vi "Core Create.vi"(8 "error in (no error)":errorcluster, 10 "Plugin Name":string, 11 "CIFTemplateNode in":refnum<class "CIFCorePlugin.lvclass">) -> (0 "error out":errorcluster, 3 "CIFTemplateNode out":refnum<class "CIFCorePlugin.lvclass">)   [LabVIEW 2021, in "CIFCorePlugin.lvclass"]
uses:
  CIFCorePlugin.lvclass
  CIFCorePlugin.lvclass/CIFCorePlugin.ctl
  CIFCoreCommon/Typedef/Plugin State.ctl
  CIFCoreCommon/CIFCoreCommon.lvlib
  CIFCoreCommon/Typedef/Timing Stats Base.ctl
  CIFCoreCommon/Typedef/Timing Statistics.ctl
  CIFCoreCommon/Typedef/FIFO Statistics.ctl
  CIFCoreCommon/Typedef/Simple Error.ctl
  CIFCoreCommon/Typedef/Monitor Doubles.ctl
  CIFCoreCommon/Typedef/Monitor U64.ctl
  CIFCoreCommon/Typedef/Monitor I64.ctl
  CIFCoreCommon/Typedef/Plugin Status.ctl
  CIFCoreCommon/Typedef/Timing Overrides.ctl
  CIFCoreCommon/Typedef/Plugin Overrides.ctl
  Typedef/Plugin Timestamps.ctl
  CIFCoreOOB/OOB_Tx/CIFCoreOOB_Tx.lvclass
  CIFCoreOOB/OOB_Rx/CIFCoreOOB_Rx.lvclass
  Typedef/Energized States.ctl
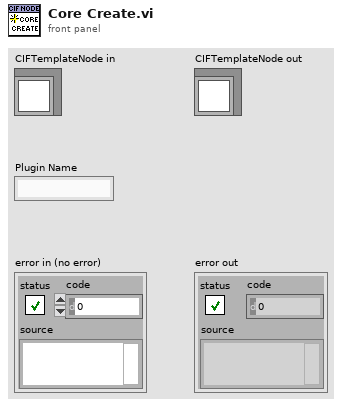
[diagram p1: front panel]
types:
  T1 = typedef "CIFCorePlugin.lvclass/Energized States.ctl" = enum16{"Prepare", "Execute", "Destroy"}
  T2 = typedef "CIFCorePlugin.lvclass/Plugin Timestamps.ctl" = enum32{"Start Creation", "Start gRPC Servers", "Start Listening", "Start Running", "Wake", "Start Execute", "Read FIFO", "Write Output", "Cycle Execute", "Start Housekeeping", "Start Sleep", "Start Cleaningup", "Start Destroying"}
  T3 = typedef "CIFCoreCommon.lvlib/Plugin Overrides.ctl" = cluster{"Timing Overrides":T4}
  T4 = typedef "CIFCoreCommon.lvlib/Timing Overrides.ctl" = cluster{"Override Timing":bool, "Period (s)":dbl}
  T5 = typedef "CIFCoreCommon.lvlib/Plugin Status.ctl" = cluster{"State":T6, "Timing Statistics (us)":T7, "FIFO Statistics (us)":T9, "error":T10, "Monitor Doubles":T11, "Monitor U64":T12, "Monitor I64":T13}
  T6 = typedef "CIFCoreCommon.lvlib/Plugin State.ctl" = enum32{"Null", "Creating", "Listening", "Running", "CleaningUp", "Destroying"}
  T7 = typedef "CIFCoreCommon.lvlib/Timing Statistics.ctl" = cluster{"Period":T8, "Wake Error":T8, "Execute":T8, "Housekeep":T8, "Idle":T8}
  T8 = typedef "CIFCoreCommon.lvlib/Timing Stats Base.ctl" = cluster{"Max":i32, "Min":i32}
  T9 = typedef "CIFCoreCommon.lvlib/FIFO Statistics.ctl" = cluster{"From T0":T8, "From Previous Plugin":T8, "Output Error":T8}
  T10 = typedef "CIFCoreCommon.lvlib/Simple Error.ctl" = cluster{"status":bool, "code":i32}
  T11 = typedef "CIFCoreCommon.lvlib/Monitor Doubles.ctl" = cluster{"1":dbl, "2":dbl, "3":dbl, "4":dbl}
  T12 = typedef "CIFCoreCommon.lvlib/Monitor U64.ctl" = cluster{"1":u64, "2":u64, "3":u64, "4":u64}
  T13 = typedef "CIFCoreCommon.lvlib/Monitor I64.ctl" = cluster{"1":i64, "2":i64, "3":i64, "4":i64}
  T14 = typedef "CIFCoreCommon.lvlib/Version.ctl" = cluster{"Major":i32, "Minor":i32, "Fix":i32, "Build":i32}
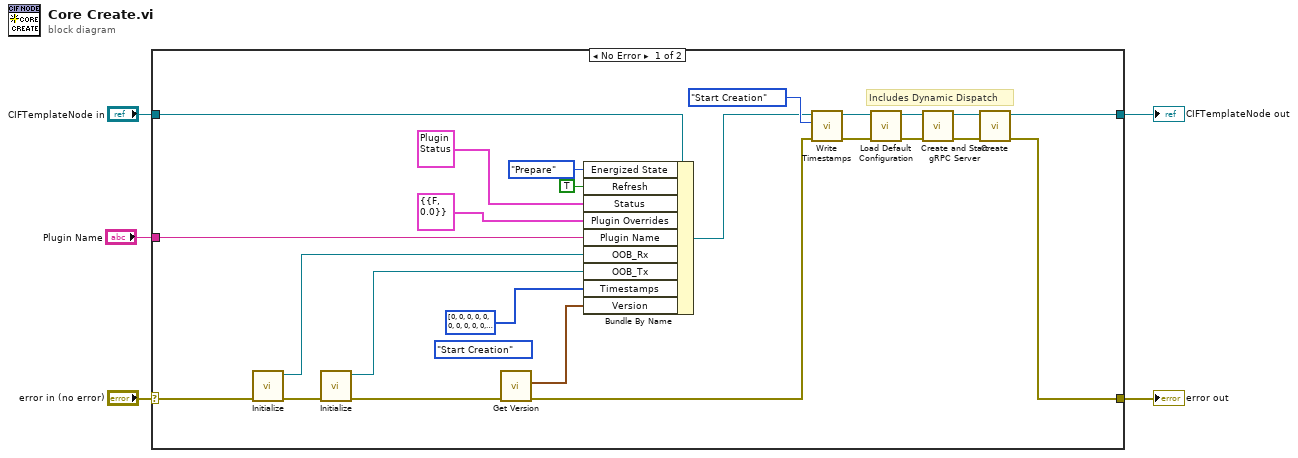
[diagram p0: block diagram]
diagram:
  n1 = case shown="No Error" "error in (no error)" {
    selector: "error in (no error)" -> [w22 w31]
    tunnel: [w9 w31] -> w4
    tunnel: [w8 w30] -> w2
    tunnel: "CIFTemplateNode in" -> [w21 w30]
    tunnel: "Plugin Name" -> [w19 _]
    frame No Error {
      (unwired) Plugin_Timestamps."Start Creation" ("Timestamps")
      # "Includes Dynamic Dispatch"
      n2 = call "Initialize.vi"("error in"=w22) -> ("error out"=w24:errorcluster, "CoreOOB_Rx out"=w26:refnum<class "CIFCoreOOB_Rx.lvclass">)  [unwired: 9 in]
      n3 = call "Initialize.vi"("error in"=w24) -> ("error out"=w18:errorcluster, "CoreOOB_Tx out"=w25:refnum<class "CIFCoreOOB_Tx.lvclass">)  [unwired: 9 in]
      n4 = call "Get Version.vi"("error in (no error)"=w18) -> ("error out"=w17:errorcluster, "Version"=w16:T14)  [unwired: 9 in]
      n5 = Bundle By Name(cluster=w21, "Energized State"=Energized_States."Prepare", "Refresh"=TRUE, "Status"=T5 {"State"=enum."Creating", "Timing Statistics (us)"={"Period"={"Max"=0, "Min"=0}, "Wake Error"={"Max"=0, "Min"=0}, "Execute"={"Max"=0, "Min"=0}, "Housekeep"={"Max"=0, "Min"=0}, "Idle"={"Max"=0, "Min"=0}}, "FIFO Statistics (us)"={"From T0"={"Max"=0, "Min"=0}, "From Previous Plugin"={"Max"=0, "Min"=0}, "Output Error"={"Max"=0, "Min"=0}}, "error"={"status"=FALSE, "code"=0}, "Monitor Doubles"={"1"=0.0, "2"=0.0, "3"=0.0, "4"=0.0}, "Monitor U64"={"1"=0, "2"=0, "3"=0, "4"=0}, "Monitor I64"={"1"=0, "2"=0, "3"=0, "4"=0}}, "Plugin Overrides"=T3 {"Timing Overrides"={"Override Timing"=FALSE, "Period (s)"=0.0}}, "Plugin Name"=w19, "OOB_Rx"=w26, "OOB_Tx"=w25, "Timestamps"=u64[] [0, 0, 0, 0, 0, 0, 0, 0, 0, 0, 0, 0, 0], "Version"=w16) -> (w20:refnum<class "CIFCorePlugin.lvclass">)
      n6 = call "Write Timestamps.vi"("error in (no error)"=w17, "Timestamp"=Plugin_Timestamps."Start Creation", "CIFTemplateNode in"=w20) -> ("error out"=w14:errorcluster, "CIFTemplateNode out"=w15:refnum<class "CIFCorePlugin.lvclass">)  [unwired: 7 in]
      n7 = call-dynamic "Load Default Configuration.vi"("error in (no error)"=w14, "CIFTemplateNode in"=w15) -> ("error out"=w13:errorcluster, "CIFTemplateNode out"=w12:refnum<class "CIFCorePlugin.lvclass">)  [unwired: 8 in]
      n8 = call "Create and Start gRPC Server.vi"("error in (no error)"=w13, "CIFTemplateNode in"=w12) -> ("error out"=w10:errorcluster, "CIFTemplateNode out"=w11:refnum<class "CIFCorePlugin.lvclass">)  [unwired: 8 in]
      n9 = call-dynamic "Create.vi"("error in (no error)"=w10, "CIFTemplateNode in"=w11) -> ("error out"=w9:errorcluster, "CIFTemplateNode out"=w8:refnum<class "CIFCorePlugin.lvclass">)  [unwired: 8 in]
    }
    frame Error {
    }
  }
  "error out" <- w4
  "CIFTemplateNode out" <- w2
